vi "SekwencjaMycia.vi"(8 "error in (no error)":errorcluster, 11 "Wash Options":T1) -> (0 "error out":errorcluster)   [LabVIEW 2020]
doc: "Author: Alex Anderson\nDate: 2/6/2013\n\nThis VI Parses a cluster of Booleans representing user selection and constructs a job\nqueue in the form of an array of clusters representing information about each job.\nThe order of array construction is important."
uses:
  controls/Station-Enum.ctl
  controls/Wash-Step-Info.ctl
  controls/WashOptions.ctl
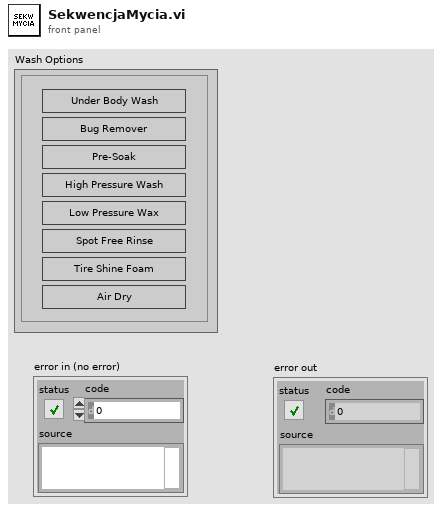
[diagram p1: front panel]
types:
  T1 = typedef "WashOptions.ctl" = cluster{"Bug Remover":bool, "Low Pressure Wax":bool, "High Pressure Wash":bool, "Pre-Soak":bool, "Spot Free Rinse":bool, "Air Dry":bool, "Under Body Wash":bool, "Tire Shine Foam":bool}
  T2 = typedef "Wash-Step-Info.ctl" = cluster{"Wash Station":T3, "Sequence Time":dbl, "Option":string}
  T3 = typedef "Station-Enum.ctl" = enum16{"Entry", "Station 1", "Station 2", "Station 3", "Exit"}
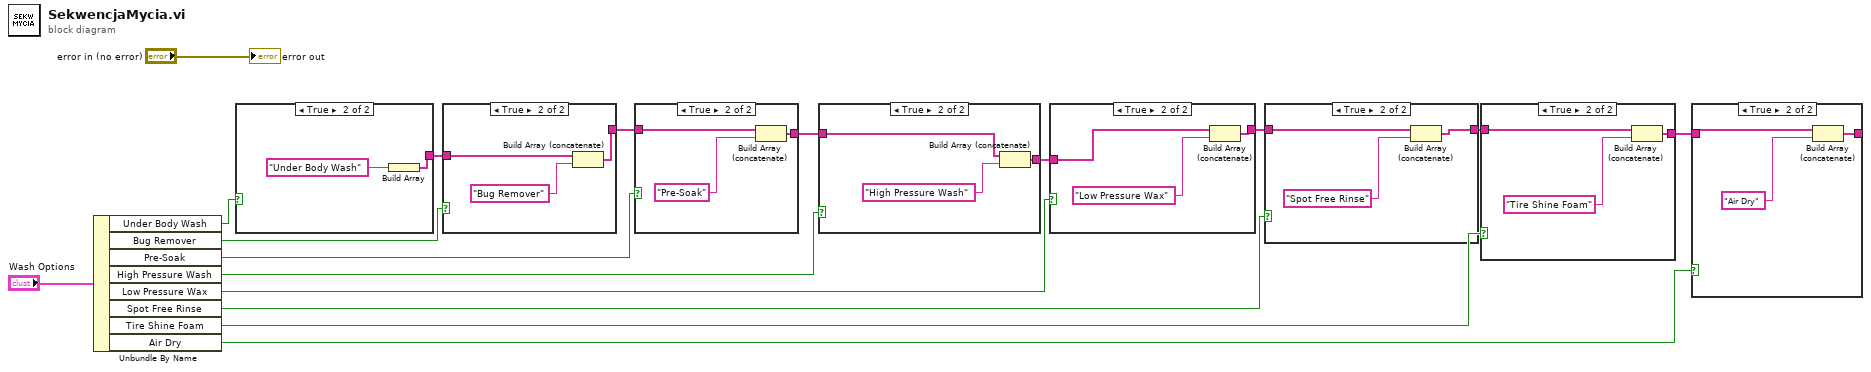
[diagram p0: block diagram]
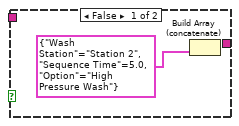
[diagram p6: hidden frame]
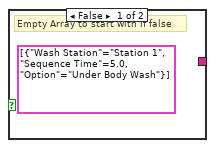
[diagram p9: hidden frame]
diagram:
  n1 = Unbundle By Name("Wash Options") -> ("Under Body Wash"=w7:bool, "Bug Remover"=w16:bool, "Pre-Soak"=w17:bool, "High Pressure Wash"=w15:bool, "Low Pressure Wax"=w14:bool, "Spot Free Rinse"=w13:bool, "Tire Shine Foam"=w12:bool, "Air Dry"=w11:bool)
  n2 = case shown="True" w7 {
    tunnel: [_ w19] -> w8
    frame False {
      w18 = T2[] [{"Wash Station"=enum."Station 1", "Sequence Time"=5.0, "Option"="Under Body Wash"}]
      # "Empty Array to start with if false"
    }
    frame True {
      n3 = Build Array("Under Body Wash") -> (w19:string[])
    }
  }
  n4 = case shown="True" w16 {
    tunnel: w8 -> [_ w22]
    tunnel: [_ w21] -> w6
    frame False {
    }
    frame True {
      n5 = Build Array (concatenate)(w22, "Bug Remover") -> (w21:string[])
    }
  }
  n6 = case shown="True" w17 {
    tunnel: w6 -> [_ w26]
    tunnel: [_ w24] -> w5
    frame False {
    }
    frame True {
      n7 = Build Array (concatenate)(w26, "Pre-Soak") -> (w24:string[])
    }
  }
  n8 = case shown="True" w15 {
    tunnel: w5 -> [_ w32]
    tunnel: [_ w30] -> w4
    frame False {
      n9 = Build Array (concatenate)(T2 {"Wash Station"=enum."Station 2", "Sequence Time"=5.0, "Option"="High Pressure Wash"}) -> (w28:T2[], w29:T2[])
    }
    frame True {
      n10 = Build Array (concatenate)(w32, "High Pressure Wash") -> (w30:string[])
    }
  }
  n11 = case shown="True" w14 {
    tunnel: w4 -> [_ w35]
    tunnel: [_ w33] -> w3
    frame False {
    }
    frame True {
      n12 = Build Array (concatenate)(w35, "Low Pressure Wax") -> (w33:string[])
    }
  }
  n13 = case shown="True" w13 {
    tunnel: w3 -> [_ w38]
    tunnel: [_ w36] -> w2
    frame False {
    }
    frame True {
      n14 = Build Array (concatenate)(w38, "Spot Free Rinse") -> (w36:string[])
    }
  }
  n15 = case shown="True" w12 {
    tunnel: w2 -> [_ w41]
    tunnel: [_ w39] -> w1
    frame False {
    }
    frame True {
      n16 = Build Array (concatenate)(w41, "Tire Shine Foam") -> (w39:string[])
    }
  }
  n17 = case shown="True" w11 {
    tunnel: w1 -> [_ w44]
    tunnel: [_ w42] -> _
    frame False {
    }
    frame True {
      n18 = Build Array (concatenate)(w44, "Air Dry") -> (w42:string[])
    }
  }
  "error out" <- "error in (no error)"
